vi "create.vi"(8 "error in (no error)":errorcluster, 10 "handle":i32) -> (0 "error out":errorcluster, 3 "Workbook":refnum<class "Workbook.lvclass">)   [LabVIEW 2020, in "Workbook.lvclass"]
uses:
  Workbook.lvclass
  Workbook.lvclass/Workbook.ctl
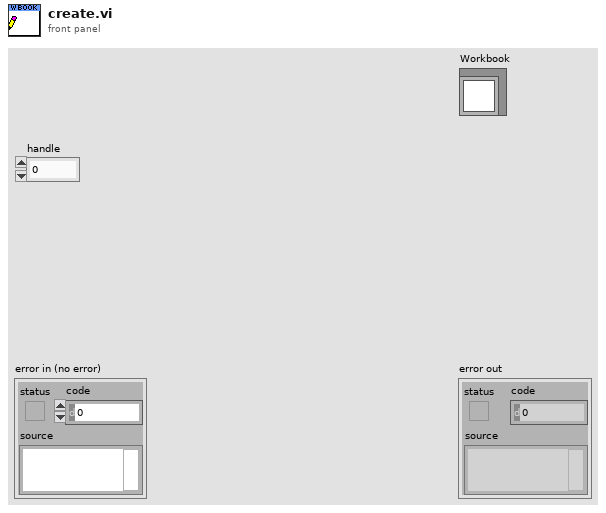
[diagram p1: front panel]
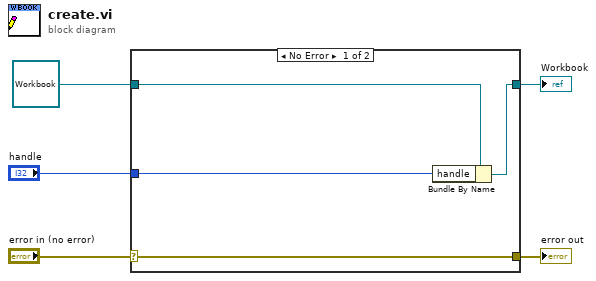
[diagram p0: block diagram]
diagram:
  n1 = case shown="No Error" "error in (no error)" {
    selector: "error in (no error)" -> [w9 w10]
    tunnel: [w9 w10] -> w4
    tunnel: [w7 w11] -> w2
    tunnel: refnum<class "Workbook.lvclass"> refnum ("Workbook in") -> [w8 w11]
    tunnel: "handle" -> [w6 _]
    frame No Error {
      n2 = Bundle By Name(cluster=w8, "handle"=w6) -> (w7:refnum<class "Workbook.lvclass">)
    }
    frame Error {
    }
  }
  "error out" <- w4
  "Workbook" <- w2
